vi "TestNewRange.vi"   [LabVIEW 2021]
uses:
  ErrorDefinitionSQLite/ErrorDefinitionSQLite.lvclass
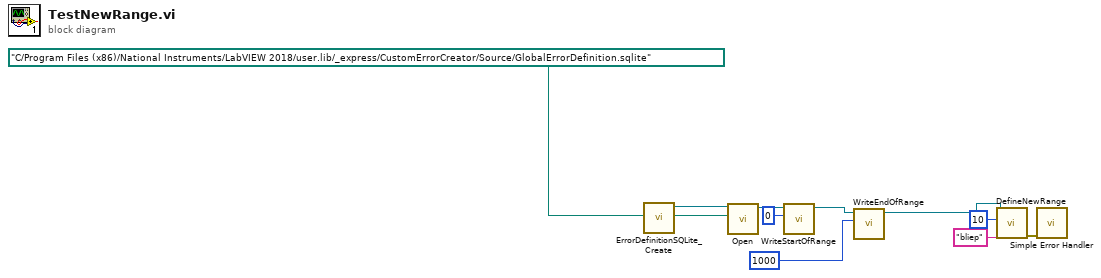
[diagram p0: block diagram]
diagram:
  n1 = call "ErrorDefinitionSQLite_Create.vi"() -> ("Reference out"=w10:refnum<class "ErrorDefinitionSQLite.lvclass">)  [unwired: 10 in, 1 out]
  n2 = call-dynamic "Open.vi"("Path"=path "C:/Program Files (x86)/National Instruments/LabVIEW 2018/user.lib/_express/CustomErrorCreator/Source/GlobalErrorDefinition.sqlite", "ReferenceIn"=w10) -> ("ReferenceOut"=w7:refnum<class "ErrorDefinitionSQLite.lvclass">)  [unwired: 8 in, 1 out]
  n3 = call-dynamic "WriteStartOfRange.vi"("StartOfRange"=0, "ReferenceIn"=w7) -> ("ReferenceOut"=w2:refnum<class "ErrorDefinitionSQLite.lvclass">)  [unwired: 8 in, 1 out]
  n4 = call-dynamic "WriteEndOfRange.vi"("MaxErrorCode"=1000, "ReferenceIn"=w2) -> ("ReferenceOut"=w6:refnum<class "ErrorDefinitionSQLite.lvclass">)  [unwired: 8 in, 1 out]
  n5 = call "DefineNewRange.vi"("LibraryName"="bliep", "RequiredSizeIn"=10 ("RequiredSize"), "DB In"=w6) -> ("ErrorOut"=w8:errorcluster)  [unwired: 7 in, 1 out]
  n6 = call <vilib>:"Simple Error Handler.vi"("error in (no error)"=w8) -> ()  [unwired: 4 in, 5 out]
